vi "Configure Master Clock Frequency.vi"(8 "error in (no error)":errorcluster, 10 "Frequency (10kHz)":u16=10 min=8 max=1000 step=1, 11 "VISA resource name":refnum<visa-resource-name>) -> (0 "error out":errorcluster, 3 "VISA resource name out":refnum<visa-resource-name>)   [LabVIEW 2021, in "Ocean Optics 2000 4000.lvlib"]
doc: "Configures the Analog to Digital Conversion Frequency to the desired value input in the VI.\n\n<B> Note: </B>\n- This VI is to be used only with the ADC1000 Analog to Digital Converter Unit\n- The Master Clock Signal is driven to twice the input frequency to meet the requirements of the S2000"
uses:
  <instrlib>/Ocean Optics 2000 4000/Ocean Optics 2000 4000.lvlib
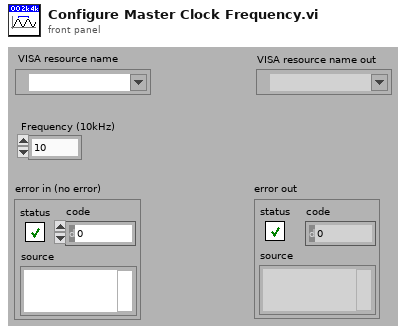
[diagram p1: front panel]
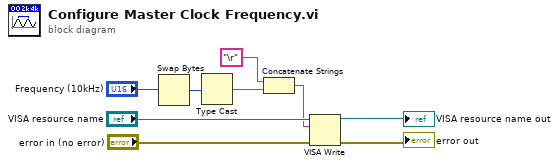
[diagram p0: block diagram]
diagram:
  n1 = Swap Bytes(anything="Frequency (10kHz)") -> (byte swapped=w5:u16)
  n2 = Type Cast(x=w5) -> (*(type *) &x=w4:string)  [unwired: 1 out]
  n3 = Concatenate Strings("\r", w4) -> (w3:string)
  n4 = VISA Write(VISA resource name="VISA resource name", write buffer=w3, error in (no error)="error in (no error)") -> (VISA resource name out=→"VISA resource name out":refnum<visa-resource-name>, error out=→"error out":errorcluster)  [unwired: 1 out]
